vi "cellularWatchdog.vi"(6 "armErrorIn":errorcluster, 8 "syringeErrorIn":errorcluster, 9 "robotPosition":i32, 10 "robotName":string, 11 "VISA Refnum in":refnum<visa-resource-name>) -> (1 "error out":errorcluster, 2 "response":string, 3 "concatenated string":string)   [LabVIEW 2021]
uses:
  Serial - Settings.ctl
  <vilib>/Instr/_visa.llb/VISA Configure Serial Port (Instr).vi
panel:
  # "Inputs"
  # "Outputs"
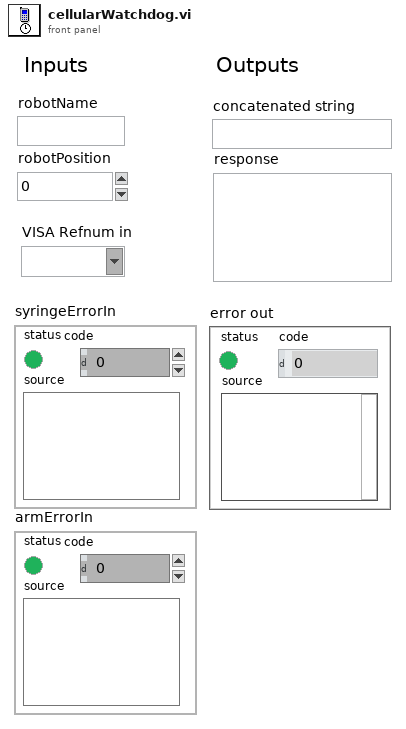
[diagram p1: front panel]
types:
  T1 = typedef "Serial - Settings.ctl" = cluster{"baud rate":u32, "data bits":u16, "parity":enum16{"None", "Odd", "Even", "Mark", "Space"}, "stop bits":u16, "flow control":u16}
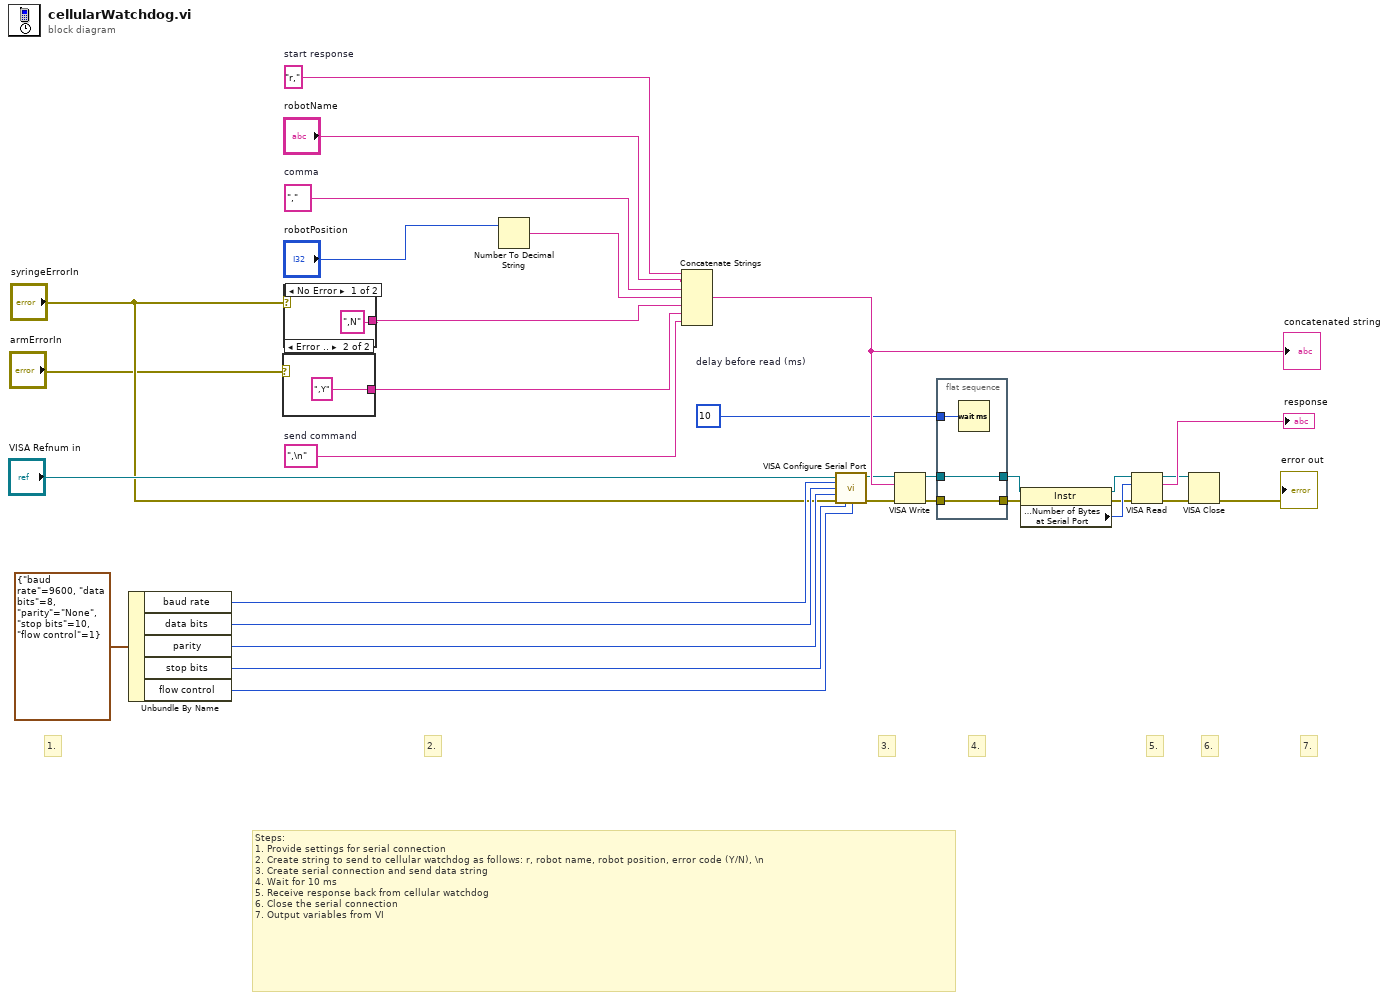
[diagram p0: block diagram]
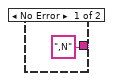
[diagram p2: hidden frame]
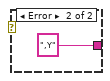
[diagram p3: hidden frame]
diagram:
  w32 = ","  # comma
  w30 = "r,"  # start response
  w3 = ",\n"  # send command
  w25 = u32 10  # delay before read (ms)
  # "Steps:\n1. Provide settings for serial connection\n2. Create string to send to cellular watchdog as follows: r, robot name, robot position, error code (Y/N), \\n\n3. Create serial connection and send data string\n4. Wait for 10 ms\n5. Receive response back from cellular watchdog\n6. Close the serial connection\n7. Output variables from VI"
  # "7."
  # "6."
  # "5."
  # "4."
  # "3."
  # "1."
  # "2."
  n1 = Unbundle By Name(T1 {"baud rate"=9600, "data bits"=8, "parity"=enum."None", "stop bits"=10, "flow control"=1} ("Serial Settings")) -> ("baud rate"=w21:u32, "data bits"=w22:u16, "parity"=w23:enum16{"None", "Odd", "Even", "Mark", "Space"}, "stop bits"=w24:u16, "flow control"=w4:u16)
  n2 = case shown="Error .." "armErrorIn" {
    tunnel: [",N" ("string") ",Y" ("string")] -> w1
    frame No Error {
    }
    frame Error {
    }
  }
  n3 = case shown="No Error" "syringeErrorIn" {
    tunnel: [",N" ("string") ",Y" ("string")] -> w5
    frame No Error {
    }
    frame Error {
    }
  }
  n4 = Number To Decimal String(number="robotPosition") -> (decimal integer string=w27:string)  [unwired: 1 in]
  n5 = Concatenate Strings(w30, "robotName", w32, w27, w5, w1, w3) -> (w29:string)
  "concatenated string" <- w29
  n6 = call-poly "VISA Configure Serial Port"("VISA resource name"="VISA Refnum in", "baud rate (9600)"=w21, "data bits (8)"=w22, "parity (0:none)"=w23, "error in (no error)"="syringeErrorIn", "stop bits (10: 1 bit)"=w24, "flow control (0:none)"=w4) -> ("VISA resource name out"=w9:refnum<visa-resource-name>, "error out"=w8:errorcluster)  [unwired: 2 in, 5 out]
  n7 = VISA Write(VISA resource name=w9, write buffer=w29, error in (no error)=w8) -> (VISA resource name out=w15:refnum<visa-resource-name>, error out=w13:errorcluster)  [unwired: 1 out]
  n8 = flat-sequence {
    tunnel: w13 -> [w38]
    tunnel: [w38] -> w14
    tunnel: w15 -> [w37]
    tunnel: [w37] -> w16
    tunnel: w25 -> [w39]
    frame #0 {
      n9 = Wait (ms)(milliseconds to wait=w39) -> ()  [unwired: 1 out]
    }
  }
  n10 = property class="Instr"(reference=w16, error in=w14) -> (reference out=w17:refnum<visa-resource-name>, error out=w18:errorcluster, "Serial Settings:Number of Bytes at Serial Port"=w20:u32)
  n11 = VISA Read(VISA resource name=w17, byte count=w20, error in (no error)=w18) -> (VISA resource name out=w11:refnum<visa-resource-name>, read buffer=→"response":string, error out=w10:errorcluster)  [unwired: 1 out]
  n12 = VISA Close(VISA resource name=w11, error in (no error)=w10) -> (error out=→"error out":errorcluster)
